vi "TSM SSC Digital PPMU Source.vi"(0 "Digital TSM In":T1, 11 "error in":errorcluster) -> (4 "Digital TSM Out":T1, 15 "error out":errorcluster)   [LabVIEW 2020]
doc: "Starts sourcing voltage or current from the PPMU on the specified pin(s) and pin group(s). This VI automatically selects the PPMU function. Changes to PPMU source settings do not take effect until you call this VI.\ns"
uses:
  TSM/TSM SSC Digital.ctl
  <vilib>/NI_TestStand_SemiconductorModule/NI_TestStand_Semiconductor_Module.lvlibp/PinMap/Digital Pattern/PinQueryContext/DigitalPatternPinQueryContext.lvclass
  SSC Digital/SSC Digital.ctl
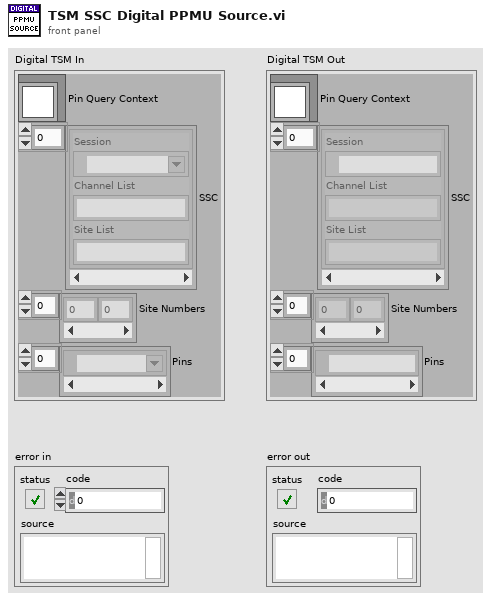
[diagram p1: front panel]
types:
  T1 = typedef "TSM SSC Digital.ctl" = cluster{"Pin Query Context":refnum<class "DigitalPatternPinQueryContext.lvclass">, "SSC":T2[], "Site Numbers":i32[], "Pins":tag[]}
  T2 = typedef "SSC Digital.ctl" = cluster{"Session":refnum<k15>, "Channel List":string, "Site List":string}
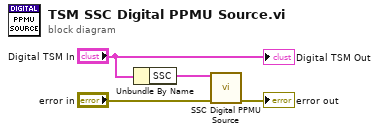
[diagram p0: block diagram]
diagram:
  n1 = Unbundle By Name("Digital TSM In") -> ("SSC"=w3:T2[])
  n2 = call "SSC Digital PPMU Source.vi"("Digital SSC in"=w3, "error in"="error in") -> ("error out"=→"error out":errorcluster)  [unwired: 12 in, 1 out]
  "Digital TSM Out" <- "Digital TSM In"
